vi "Set channel parameters.vi"(8 "error in (no error)":errorcluster, 11 "Channel Rep in":refnum<class "Channel Rep.lvclass">) -> (0 "error out":errorcluster, 3 "Channel Rep out":refnum<class "Channel Rep.lvclass">)   [LabVIEW 2018, in "Channel Rep.lvclass"]
uses:
  Channel Rep.lvclass
  <vilib>/addons/zeromq/socket_type.ctl
  Socket/Socket.lvclass
  <vilib>/addons/zeromq/zeromq.lvlib
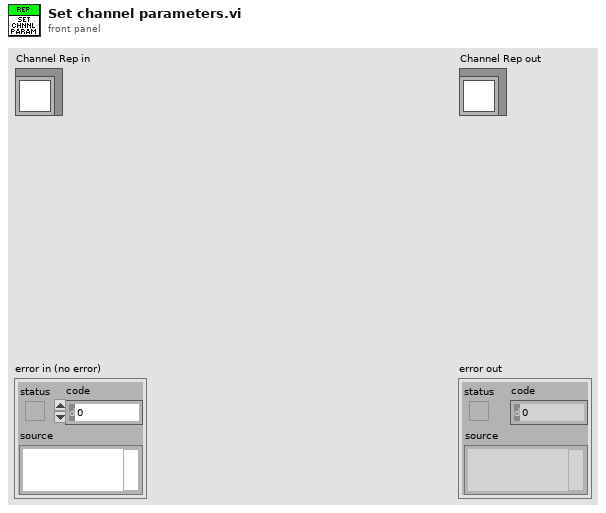
[diagram p1: front panel]
types:
  T1 = typedef "zeromq.lvlib/socket_type.ctl" = enum8{"ZMQ_PAIR", "ZMQ_PUB", "ZMQ_SUB", "ZMQ_REQ", "ZMQ_REP", "ZMQ_DEALER", "ZMQ_ROUTER", "ZMQ_PULL", "ZMQ_PUSH", "ZMQ_XPUB", "ZMQ_XSUB", "ZMQ_STREAM", "ZMQ_SERVER", "ZMQ_CLIENT", "ZMQ_RADIO", "ZMQ_DISH", "ZMQ_GATHER", "ZMQ_SCATTER", "ZMQ_DGRAM"}
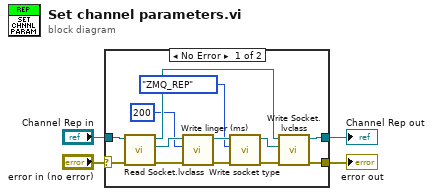
[diagram p0: block diagram]
diagram:
  n1 = case shown="No Error" "error in (no error)" {
    selector: "error in (no error)" -> [w16 w18]
    tunnel: "Channel Rep in" -> [w17 w19]
    tunnel: [w14 w19] -> w2
    tunnel: [w13 w18] -> w1
    frame No Error {
      n2 = call-dynamic "Read Socket.lvclass.vi"("error in (no error)"=w16, "Communication Channel in"=w17) -> ("error out"=w7:errorcluster, "Socket.lvclass"=w12:refnum<class "Socket.lvclass">, "Communication Channel out"=w15:refnum<class "Channel Rep.lvclass">)  [unwired: 7 in]
      n3 = call-dynamic "Write linger (ms).vi"("error in (no error)"=w7, "linger (ms)"=200, "Socket in"=w12) -> ("error out"=w8:errorcluster, "Socket out"=w11:refnum<class "Socket.lvclass">)  [unwired: 7 in]
      n4 = call-dynamic "Write socket type.vi"("error in (no error)"=w8, "Socket type"=socket_type."ZMQ_REP", "Socket in"=w11) -> ("error out"=w9:errorcluster, "Socket out"=w10:refnum<class "Socket.lvclass">)  [unwired: 7 in]
      n5 = call-dynamic "Write Socket.lvclass.vi"("error in (no error)"=w9, "Socket2.lvclass"=w10, "Communication Channel in"=w15) -> ("error out"=w13:errorcluster, "Communication Channel out"=w14:refnum<class "Channel Rep.lvclass">)  [unwired: 7 in]
    }
    frame Error {
    }
  }
  "error out" <- w1
  "Channel Rep out" <- w2
